vi "生成消息.vi"(9 "值":sgl, 10 "属性":enum16{"温度", "亮度", "电量", "连接质量"}(ring), 11 "节点ID":i32=1) -> (3 "输出簇":T1)   [LabVIEW 2012]
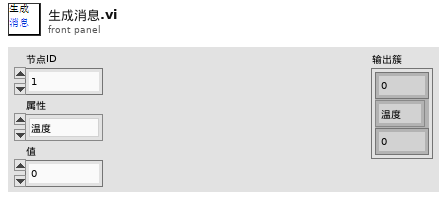
[diagram p1: front panel]
types:
  T1 = cluster{i32, enum16{"温度", "亮度", "电量", "连接质量"}, sgl}
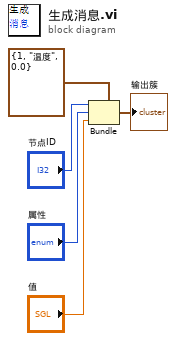
[diagram p0: block diagram]
diagram:
  n1 = Bundle(cluster=T1 {1, enum."温度", 0.0}, "节点ID", "属性", "值") -> (→"输出簇":T1)
